vi "WS1050 RFFE Write Read Updated.vi"(0 "VISA resource name":refnum<visa-resource-name>="COM1", 1 "write buffer":string, 2 "delay before read (ms)":u32=100, 3 "error in (no error)":errorcluster) -> (6 "VISA resource name out":refnum<visa-resource-name>, 7 "EFuse Read Back":string, 10 "error out":errorcluster)   [LabVIEW 2012]
doc: "The Basic Serial Read and Write example performs a Serial Port Read, a Serial Port Write, or a combination of these actions. The user selects the actions (read or write) on the front panel. If both are selected, the VI will write the data first, read data, and then close the VISA session that is opened to the port. This VI will wait until the specified number of bytes is received at the port. Only the number of bytes specified will be read.\n\nINSTRUCTIONS:\n1) Select the serial resource and configuration parameters (baud rate, data bits, parity, stop bits, flow control).\n2) Select the operations to be performed. \n3) Connect the serial port to your device. If no device is available, perform a loopback test by doing one of the following. Short pins 2 and 3 on a RS-232 cable or short pin 4 to pin 8 and pin 5 to pin 9 on a RS-485/422 cable. \n4) Run the VI to see the data read. (The \"read string\" will match the \"string to write\" if a loopback test was performed.)\n\nNote: The parameters set for the serial port must match the parameters of the connected instrument or device. In this example, the bytes to read parameter specifies the number of bytes that the serial port reads. If there were more bytes at the port than the number specified in bytes to read, those bytes would not be read. Also, if you specify to read more bytes than the number of bytes actually read, you might receive a timeout error message.\n\nOn the block diagram, the Configure Serial Port VI sets the configuration parameters. The front panel displays the controls used to configure the basic parameters, such as baud rate, data bits, and parity. Constants configure the other parameters the user probably does not need set. After the VISA Configure Serial Port VI opens the VISA session and configures the port, the VI passes the VISA resource name to other VIs that perform operations on that VISA resource. The VISA Write function sends a command to the serial device and the VISA Read function returns data based on the command. The VISA Close function then closes the reference to the serial device. It is important to close the reference; otherwise communication through with that port through protocols other than VISA might not be possible."
panel:
  out "read buffer":string
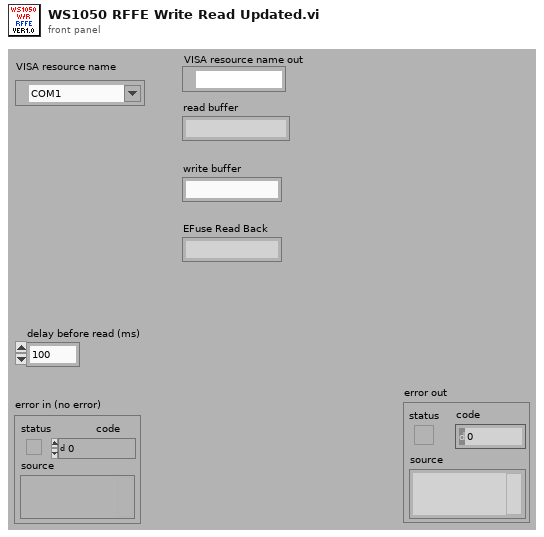
[diagram p1: front panel]
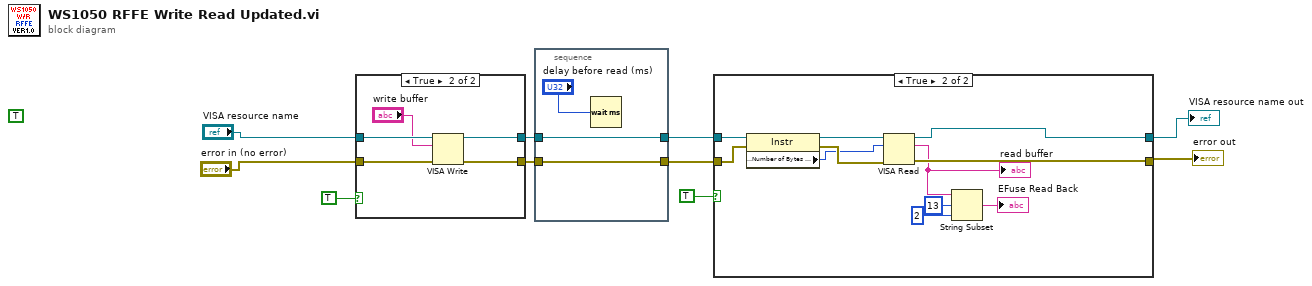
[diagram p0: block diagram]
diagram:
  (unwired) TRUE
  n1 = case shown="True" TRUE {
    tunnel: [w12 w17] -> w10
    tunnel: "VISA resource name" -> [w11 w16]
    tunnel: "error in (no error)" -> [w12 w15]
    tunnel: [w11 w14] -> w8
    frame False {
    }
    frame True {
      n2 = VISA Write(VISA resource name=w16, write buffer="write buffer", error in (no error)=w15) -> (VISA resource name out=w14:refnum<visa-resource-name>, error out=w17:errorcluster)  [unwired: 1 out]
    }
  }
  n3 = stacked-sequence {
    tunnel: w10 -> [w20]
    tunnel: [w20] -> w9
    tunnel: w8 -> [w19]
    tunnel: [w19] -> w7
    frame #0 {
      n4 = Wait (ms)(milliseconds to wait="delay before read (ms)") -> ()  [unwired: 1 out]
    }
  }
  n5 = case shown="True" TRUE {
    tunnel: w9 -> [w22 w31]
    tunnel: [w22 w24] -> w1
    tunnel: [w21 w25] -> w5
    tunnel: w7 -> [w21 w33]
    frame False {
    }
    frame True {
      n6 = property class="Instr"(reference=w33, error in=w31) -> (reference out=w32:refnum<visa-resource-name>, error out=w30:errorcluster, "Serial Settings:Number of Bytes at Serial Port"=w28:u32)
      n7 = VISA Read(VISA resource name=w32, byte count=w28, error in (no error)=w30) -> (VISA resource name out=w25:refnum<visa-resource-name>, read buffer=w23:string, error out=w24:errorcluster)  [unwired: 1 out]
      "read buffer" <- w23
      n8 = String Subset(string=w23, offset (0)=13, length (rest)=2 ("length (rest)")) -> (substring=→"EFuse Read Back":string)
    }
  }
  "error out" <- w1
  "VISA resource name out" <- w5
